vi "Doe_Julabo_Control.vi"(0 "Julabo CF41 VISA":refnum<visa-resource-name>="COM3", 1 "Data Cluster In":T1={"Current DoE"=[], "SSI 1 Flow Rate"=0.0, "SSI 2 Flow Rate"=0.0, "FLOM 1 Flow Rate"=0.0, "FLOM 2 Flow Rate"=0.0, "Pumps Running?"=FALSE, "Boolean 2"=FALSE, "Boolean 3"=FALSE, "Boolean 4"=FALSE, "At Equilibrium?"=FALSE, "Script Running?"=FALSE, "Current Script Iteration"=0.0, "Total Script Iterations"=0.0, "FLOM Pumps VISA"="COM2", "SSI 1 Pump VISA"="COM76", "SSI 2 Pump VISA"="COM74", "Huber Unistat VISA"="COM1", "SSI 3 Pump VISA"="COM76", "SSI 4 Pump VISA"="COM76", "SSI 4 Flow Rate"=0.0, "SSI 3 Flow Rate"=0.0, "Flow Meter 1 Rate "=0.0, "Flow Meter 2 Rate"=0.0, "Flow Meter 3 Rate"=0.0, "Flow Meter 4 Rate"=0.0, "SSI 1 Flow Setpoint"=0.0, "SSI 2 Flow Setpoint"=0.0, "SSI 3 Flow Setpoint"=0.0, "SSI 4 Flow Setpoint"=0.0, "Temperature Setpoint"=0.0, "Flow meter 3 COM"=17, "Flow meter 5 COM"=18, "Flow meter 4 COM"=19, "Flow meter 2 COM"=16, "Flow meter 1 COM"=15, "Unit"=enum."PSI", "Pressure COM"="COM6", "Julabo Setpoint"=0.0, "Julabo Control"=enum."Internal", "Overtemp"=50.0, "Subtemp"=-20.0, "HeatMax"=50, "CoolMax"=-100, "InternMax"=50.0, "InternMin"=0.0, "Upper Bandlimit"=100.0, "Lower Bandlimit"=0.0, "Julabo CF41 VISA"="COM3", "Xp (0.6K) Int"=0.6, "Tn (3s) Int"=3, "Tv (0s) Int"=0, "Dynamic (0: aperiodic) Int"=enum."aperiodic", "Xp (0.6K) Ext"=0.6, "Tn (3s) Ext"=3, "Tv (0s) Ext"=0, "XpU (0.6K) Ext"=0.6} {"XpU (0.6K) Ext" min=0.1 max=99.9; "Tv (0s) Ext" max=999; "Tn (3s) Ext" min=3 max=9999; "Xp (0.6K) Ext" min=0.1 max=99.9; "Tv (0s) Int" max=999; "Tn (3s) Int" min=3 max=9999; "Xp (0.6K) Int" min=0.1 max=99.9; "Lower Bandlimit" min=0.0 max=200.0; "Upper Bandlimit" min=0.0 max=200.0; "InternMin" format="%.2f"; "InternMax" format="%.2f"; "CoolMax" min=-100 max=0; "HeatMax" max=100; "Subtemp" format="%.2f"; "Overtemp" format="%.2f"; "Julabo Setpoint" format="%.2f"; "Current DoE" format="%0.3f"}, 5 "Serial Configuration":T4={"Baud Rate"=4800, "Parity"=2, "Data Bits"=7, "Stop Bits"=10, "Flow Control"=2} {"Flow Control" items=["None", "XON/XOFF", "RTS/CTS", "XON/XOFF & RTS/CTS", "DTR/DSR", "XON/XOFF & DTR/DSR"]; "Stop Bits" items=["1.0"=10, "1.5"=15, "2.0"=20]; "Data Bits" items=["7"=7, "8"=8]; "Parity" items=["None", "Odd", "Even", "Mark", "Space"]; "Baud Rate" items=["300"=300, "600"=600, "1200"=1200, "2400"=2400, "4800"=4800, "9600"=9600, "19200"=19200]}, 7 "RS485-Address (128: RS232)":u32=128, 9 "ID Query? (T: Yes)":bool=TRUE, 11 "ReadCycle":i32=1000) -> (4 "Data Cluster Out":T1={"Current DoE"=[], "SSI 1 Flow Rate"=0.0, "SSI 2 Flow Rate"=0.0, "FLOM 1 Flow Rate"=0.0, "FLOM 2 Flow Rate"=0.0, "Pumps Running?"=FALSE, "Boolean 2"=FALSE, "Boolean 3"=FALSE, "Boolean 4"=FALSE, "At Equilibrium?"=FALSE, "Script Running?"=FALSE, "Current Script Iteration"=0.0, "Total Script Iterations"=0.0, "FLOM Pumps VISA"="COM2", "SSI 1 Pump VISA"="COM76", "SSI 2 Pump VISA"="COM74", "Huber Unistat VISA"="COM1", "SSI 3 Pump VISA"="COM76", "SSI 4 Pump VISA"="COM76", "SSI 4 Flow Rate"=0.0, "SSI 3 Flow Rate"=0.0, "Flow Meter 1 Rate "=0.0, "Flow Meter 2 Rate"=0.0, "Flow Meter 3 Rate"=0.0, "Flow Meter 4 Rate"=0.0, "SSI 1 Flow Setpoint"=0.0, "SSI 2 Flow Setpoint"=0.0, "SSI 3 Flow Setpoint"=0.0, "SSI 4 Flow Setpoint"=0.0, "Temperature Setpoint"=0.0, "Flow meter 3 COM"=17, "Flow meter 5 COM"=18, "Flow meter 4 COM"=19, "Flow meter 2 COM"=16, "Flow meter 1 COM"=15, "Unit"=enum."PSI", "Pressure COM"="COM6", "Julabo Setpoint"=0.0, "Julabo Control"=enum."Internal", "Overtemp"=50.0, "Subtemp"=-20.0, "HeatMax"=50, "CoolMax"=-100, "InternMax"=50.0, "InternMin"=0.0, "Upper Bandlimit"=100.0, "Lower Bandlimit"=0.0, "Julabo CF41 VISA"="COM3", "Xp (0.6K) Int"=0.6, "Tn (3s) Int"=3, "Tv (0s) Int"=0, "Dynamic (0: aperiodic) Int"=enum."aperiodic", "Xp (0.6K) Ext"=0.6, "Tn (3s) Ext"=3, "Tv (0s) Ext"=0, "XpU (0.6K) Ext"=0.6} {"XpU (0.6K) Ext" min=0.1 max=99.9; "Tv (0s) Ext" max=999; "Tn (3s) Ext" min=3 max=9999; "Xp (0.6K) Ext" min=0.1 max=99.9; "Tv (0s) Int" max=999; "Tn (3s) Int" min=3 max=9999; "Xp (0.6K) Int" min=0.1 max=99.9; "Lower Bandlimit" min=0.0 max=200.0; "Upper Bandlimit" min=0.0 max=200.0; "InternMin" format="%.2f"; "InternMax" format="%.2f"; "CoolMax" min=-100 max=0; "HeatMax" max=100; "Subtemp" format="%.2f"; "Overtemp" format="%.2f"; "Julabo Setpoint" format="%.2f"; "Current DoE" format="%0.3f"}, 6 "Internal Temp":dbl format="%.2f", 8 "External Temp":dbl format="%.2f", 15 "device error out":errorcluster)   [LabVIEW 2015, in "JULABO DeviceDriver.lvlib"]
doc: "Advanced event triggered example"
uses:
  <instrlib>/JULABO DeviceDriver/JULABO DeviceDriver.lvlib
  <instrlib>/JULABO DeviceDriver/Examples/Julabo Serial Control.ctl
  --Controls and TypeDefs--/DoE_Control_Cluster.ctl
panel:
  out "error out 2":errorcluster caption="error out"
  out "error out":errorcluster
  in  "Registerkartenelement":T2(tab)
  out "Safety Temp":dbl
  out "Excess Temp Protection":dbl
  in  "Control":enum16{"Internal", "External"}(ring)
  in  "Setpoint":dbl format="%.2f"
  out "Power":i8(slide) scale=-100.0..100.0
  out "Diagram":T3(graph)
  in  "StartStop":bool
  in  "btnAdjustInternalTempLimits":bool
  in  "btnAdjustBandLimits":bool
  in  "btnAdjustCapacityLevels":bool
  in  "btnAdjustWarningLevels":bool
  in  "Upper Bandlimit":dbl=100.0 min=0.0 max=200.0
  in  "Lower Bandlimit":dbl min=0.0 max=200.0
  in  "InternMin":dbl format="%.2f"
  in  "InternMax":dbl=50.0 format="%.2f"
  in  "CoolMax":i8=-100 min=-100 max=0
  in  "HeatMax":u8=50 max=100
  in  "Subtemp":dbl=-20.0 format="%.2f"
  in  "Overtemp":dbl=50.0 format="%.2f"
  in  "Tv (0s) 2":u16 max=999
  in  "Tn (3s) 2":u16=3 min=3 max=9999
  in  "Xp (0.6K) 2":dbl=0.6 min=0.1 max=99.9
  in  "btnAdjustExternalControlParams":bool
  in  "XpU (0.6K)":dbl=0.6 min=0.1 max=99.9
  in  "Dynamic (0: aperiodic)":enum16{"aperiodic", "standard"}(ring)
  in  "btnAdjustInternalControlParams":bool
  in  "Tv (0s)":u16 max=999
  in  "Tn (3s)":u16=3 min=3 max=9999
  in  "Xp (0.6K)":dbl=0.6 min=0.1 max=99.9
  in  "Stopp":bool
  in  "Reset / Default (T: Both)":bool=TRUE
  # "1. Select the COM-Port and adjust the serial\nconfiguration for your instrument\n2. Adjust the Read cycle\n3. Start the VI by pressing the \"Start\" -Button\n( Arrow button on the top-left corner)\n4. To stop the execution press the \"Stop\" button"
  # "Julabo"
  # "Limits"
  # "PID Control Parameters"
  # "Julabo"
  # "Limits"
  # "PID Control Parameters"
  # "Internal parameters"
  # "External parameters"
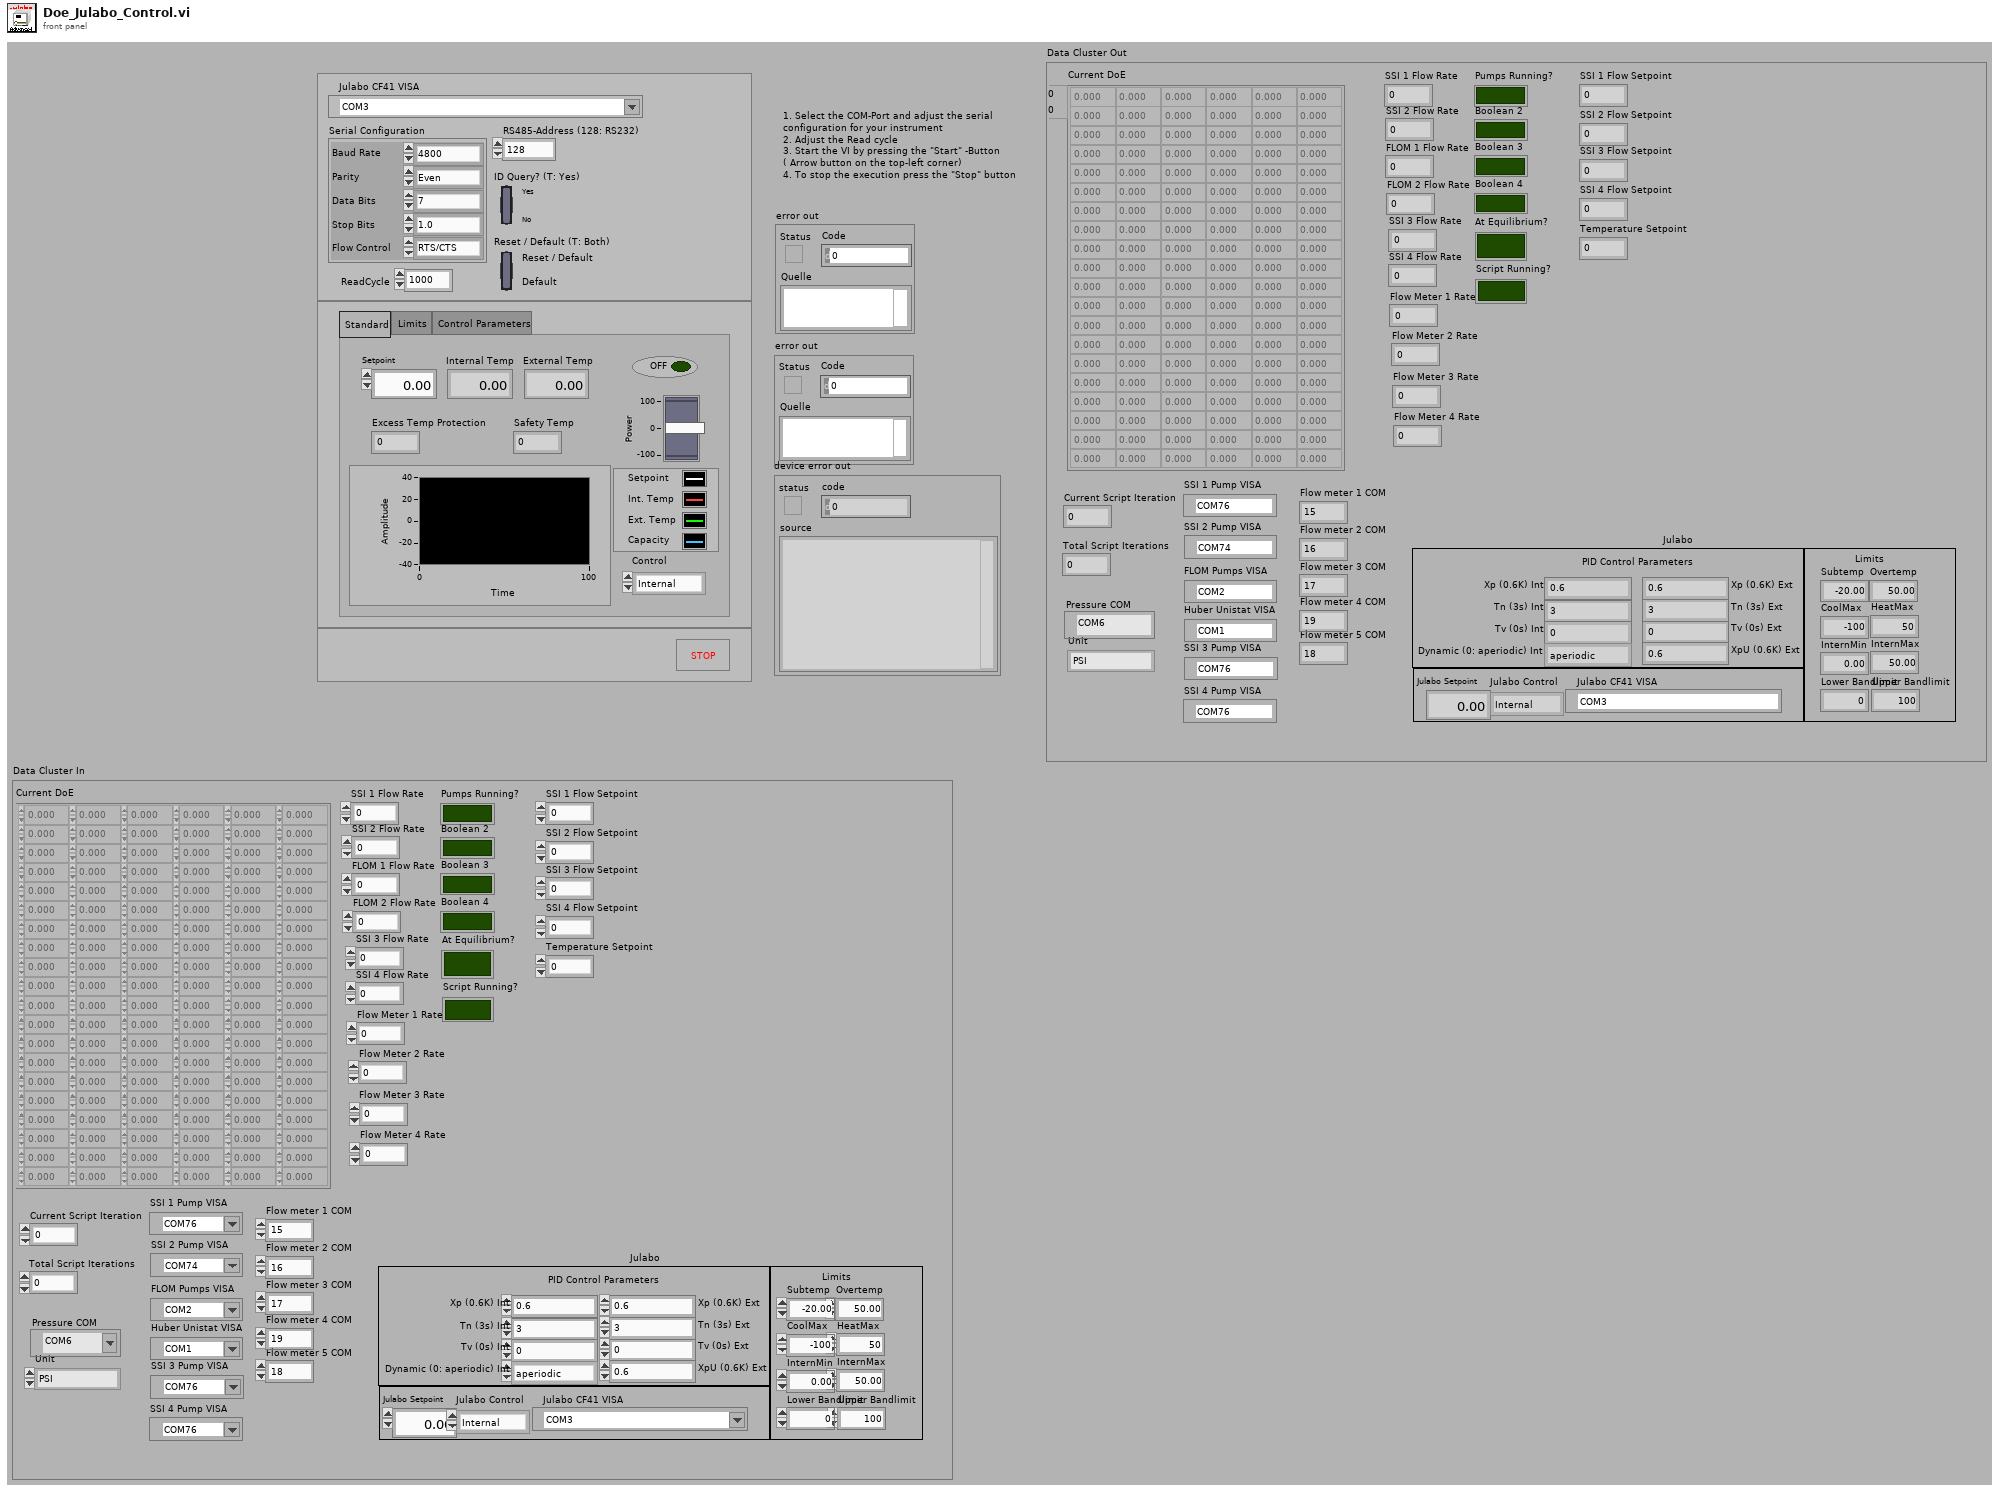
[diagram p1: front panel]
types:
  T1 = typedef "DoE_Control_Cluster.ctl" = cluster{"Current DoE":dbl[][], "SSI 1 Flow Rate":dbl, "SSI 2 Flow Rate":dbl, "FLOM 1 Flow Rate":dbl, "FLOM 2 Flow Rate":dbl, "Pumps Running?":bool, "Boolean 2":bool, "Boolean 3":bool, "Boolean 4":bool, "At Equilibrium?":bool, "Script Running?":bool, "Current Script Iteration":dbl, "Total Script Iterations":dbl, "FLOM Pumps VISA":refnum<visa-resource-name>, "SSI 1 Pump VISA":refnum<visa-resource-name>, "SSI 2 Pump VISA":refnum<visa-resource-name>, "Huber Unistat VISA":refnum<visa-resource-name>, "SSI 3 Pump VISA":refnum<visa-resource-name>, "SSI 4 Pump VISA":refnum<visa-resource-name>, "SSI 4 Flow Rate":dbl, "SSI 3 Flow Rate":dbl, "Flow Meter 1 Rate ":dbl, "Flow Meter 2 Rate":dbl, "Flow Meter 3 Rate":dbl, "Flow Meter 4 Rate":dbl, "SSI 1 Flow Setpoint":dbl, "SSI 2 Flow Setpoint":dbl, "SSI 3 Flow Setpoint":dbl, "SSI 4 Flow Setpoint":dbl, "Temperature Setpoint":dbl, "Flow meter 3 COM":u16, "Flow meter 5 COM":u16, "Flow meter 4 COM":u16, "Flow meter 2 COM":u16, "Flow meter 1 COM":u16, "Unit":enum16{"PSI", "Bar", "cm H2O", "ft H2O", "hectoPascal", "in Hg", "in H2O", "kiloPascal", "milliBar", "mmHg", "MegaPascal", "Numeric Pressure"}, "Pressure COM":refnum<visa-resource-name>, "Julabo Setpoint":dbl, "Julabo Control":enum16{"Internal", "External"}, "Overtemp":dbl, "Subtemp":dbl, "HeatMax":u8, "CoolMax":i8, "InternMax":dbl, "InternMin":dbl, "Upper Bandlimit":dbl, "Lower Bandlimit":dbl, "Julabo CF41 VISA":refnum<visa-resource-name>, "Xp (0.6K) Int":dbl, "Tn (3s) Int":u16, "Tv (0s) Int":u16, "Dynamic (0: aperiodic) Int":enum16{"aperiodic", "standard"}, "Xp (0.6K) Ext":dbl, "Tn (3s) Ext":u16, "Tv (0s) Ext":u16, "XpU (0.6K) Ext":dbl}
  T2 = enum32{"Standard", "Limits", "Control Parameters"}
  T3 = cluster{"Setpoint (out)":dbl, "InternalTemp (out)":dbl, "ExternalTemp (out)":dbl, "Capacity (out)":i8}
  T4 = typedef "Julabo Serial Control.ctl" = cluster{"Baud Rate":u32, "Parity":u16, "Data Bits":u16, "Stop Bits":u16, "Flow Control":u16}
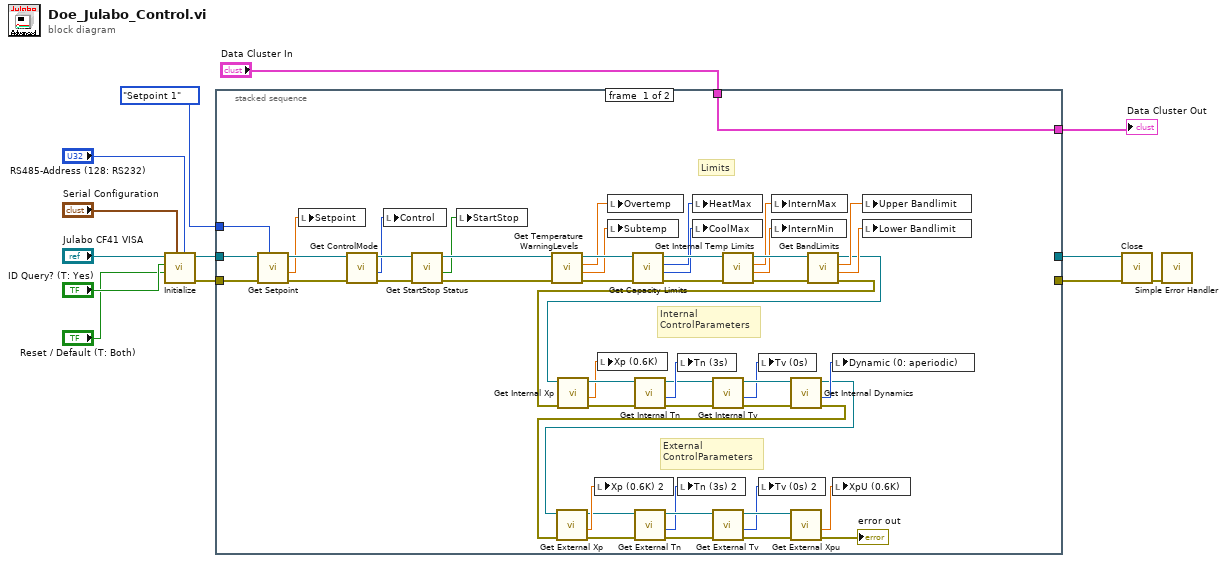
[diagram p0: block diagram]
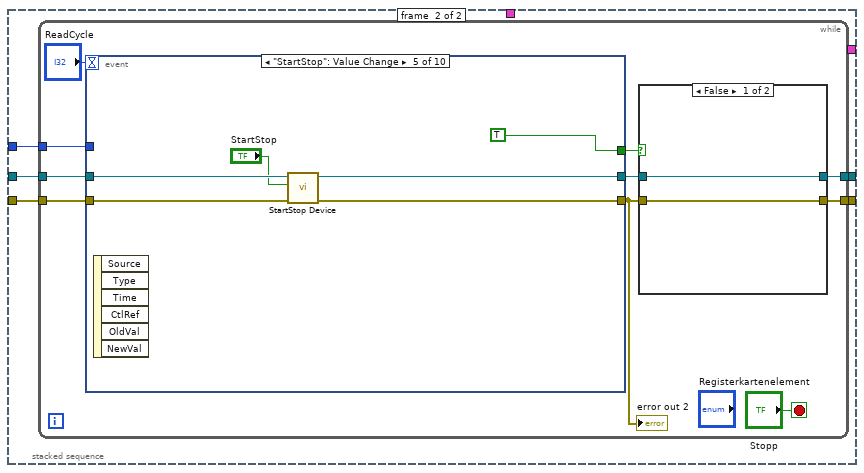
[diagram p2: hidden frame]
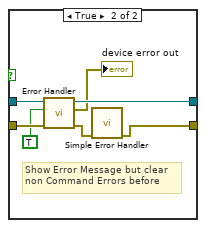
[diagram p3: hidden frame]
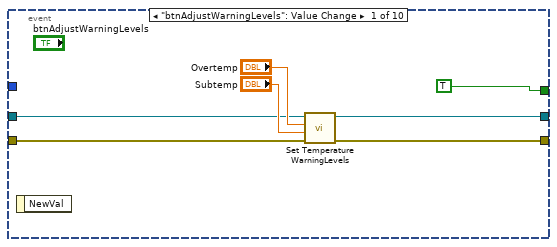
[diagram p4: hidden frame]
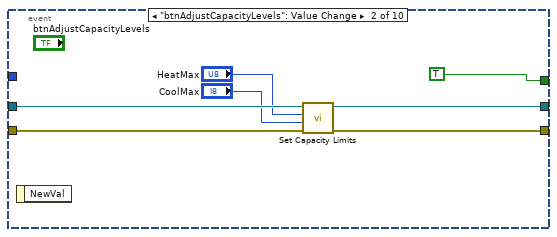
[diagram p5: hidden frame]
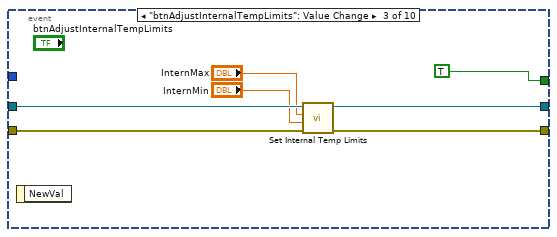
[diagram p6: hidden frame]
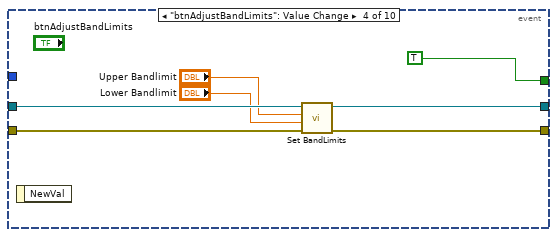
[diagram p7: hidden frame]
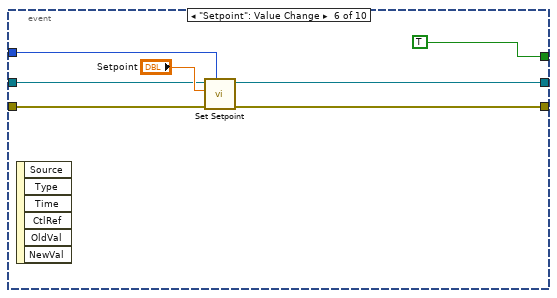
[diagram p8: hidden frame]
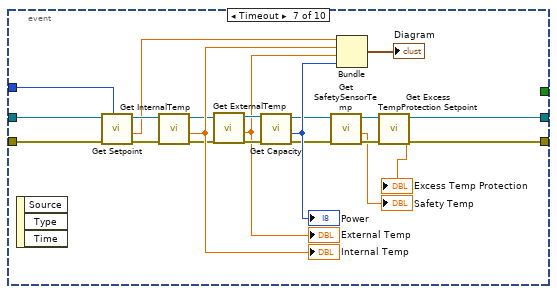
[diagram p9: hidden frame]
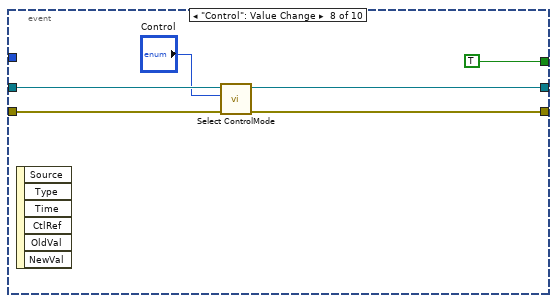
[diagram p10: hidden frame]
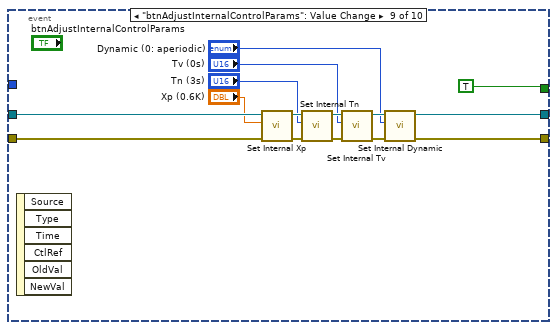
[diagram p11: hidden frame]
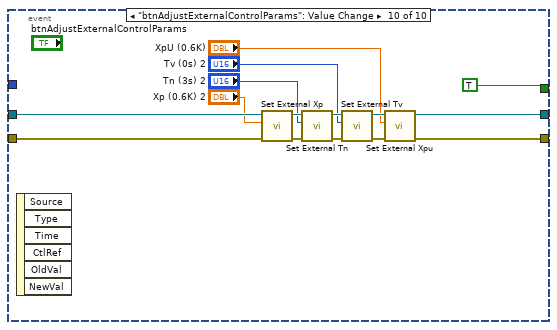
[diagram p12: hidden frame]
diagram:
  n1 = call <instrlib>:"Initialize.vi"("RS485-Address (128: RS232)"="RS485-Address (128: RS232)", "Serial Configuration"="Serial Configuration", "Reset / Default (T: Both)"="Reset / Default (T: Both)", "ID Query? (T: Yes)"="ID Query? (T: Yes)", "VISA resource name"="Julabo CF41 VISA") -> ("error out"=w6:errorcluster, "VISA resource name out"=w7:refnum<visa-resource-name>)  [unwired: 5 in]
  n2 = stacked-sequence {
    tunnel: w7 -> [w20 w70]
    tunnel: w6 -> [w19 w69]
    tunnel: [_ w68] -> w5
    tunnel: [_ w67] -> w4
    tunnel: enum16{"Setpoint 1", "Setpoint 2", "Setpoint 3"}."Setpoint 1" ("Setpointindex") -> [w16 w66]
    tunnel: "Data Cluster In" -> [w14 _]
    tunnel: [w14 _] -> w1
    frame #0 {
      # "External\nControlParameters"
      # "Internal\nControlParameters"
      # "Limits"
      n3 = call <instrlib>:"Get Setpoint.vi"("Setpointindex"=w16, "error in (no error)"=w19, "VISA resource name"=w20) -> ("error out"=w17:errorcluster, "Setpoint (out)"=w15:dbl, "VISA resource name out"=w18:refnum<visa-resource-name>)  [unwired: 6 in]
      n4 = local write "Setpoint"(w15) -> ()
      n5 = call <instrlib>:"Get ControlMode.vi"("error in"=w17, "VISA resource name in"=w18) -> ("error out"=w22:errorcluster, "Control (out)"=w26:enum16{"Internal", "External"}, "VISA resource name out"=w27:refnum<visa-resource-name>)  [unwired: 7 in]
      n6 = local write "Control"(w26) -> ()
      n7 = call <instrlib>:"Get StartStop Status.vi"("error in"=w22, "VISA resource name in"=w27) -> ("error out"=w21:errorcluster, "Status"=w23:bool, "VISA resource name out"=w24:refnum<visa-resource-name>)  [unwired: 7 in]
      n8 = local write "StartStop"(w23) -> ()
      n9 = call <instrlib>:"Get Temperature WarningLevels.vi"("error in (no error)"=w21, "VISA resource name"=w24) -> ("error out"=w62:errorcluster, "Subtemp (out)"=w53:dbl, "Overtemp (out)"=w52:dbl, "VISA resource name out"=w65:refnum<visa-resource-name>)  [unwired: 2 in]
      n10 = local write "Overtemp"(w52) -> ()
      n11 = local write "Subtemp"(w53) -> ()
      n12 = call <instrlib>:"Get Capacity Limits.vi"("error in (no error)"=w62, "VISA resource name"=w65) -> ("error out"=w61:errorcluster, "Maximum cooling capacity(out)"=w55:i8, "Maximum heating capacity(out)"=w54:u8, "VISA resource name out"=w64:refnum<visa-resource-name>)  [unwired: 2 in]
      n13 = local write "HeatMax"(w54) -> ()
      n14 = local write "CoolMax"(w55) -> ()
      n15 = call <instrlib>:"Get Internal Temp Limits.vi"("error in (no error)"=w61, "VISA resource name"=w64) -> ("error out"=w60:errorcluster, "IntMin (out)"=w57:dbl, "IntMax (out)"=w56:dbl, "VISA resource name out"=w63:refnum<visa-resource-name>)  [unwired: 2 in]
      n16 = local write "InternMax"(w56) -> ()
      n17 = local write "InternMin"(w57) -> ()
      n18 = call <instrlib>:"Get BandLimits.vi"("error in (no error)"=w60, "VISA resource name"=w63) -> ("error out"=w40:errorcluster, "LowerBand (out)"=w59:dbl, "UpperBand (out)"=w58:dbl, "VISA resource name out"=w41:refnum<visa-resource-name>)  [unwired: 2 in]
      n19 = call <instrlib>:"Get Internal Xp.vi"("error in"=w40, "VISA resource name in"=w41) -> ("error out"=w43:errorcluster, "InternalXp (out)"=w42:dbl, "VISA resource name out"=w44:refnum<visa-resource-name>)  [unwired: 7 in]
      n20 = local write "Xp (0.6K)"(w42) -> ()
      n21 = call <instrlib>:"Get Internal Tn.vi"("error in"=w43, "VISA resource name in"=w44) -> ("error out"=w45:errorcluster, "InternalTn (out)"=w51:u16, "VISA resource name out"=w46:refnum<visa-resource-name>)  [unwired: 7 in]
      n22 = local write "Tn (3s)"(w51) -> ()
      n23 = call <instrlib>:"Get Internal Tv.vi"("error in"=w45, "VISA resource name in"=w46) -> ("error out"=w48:errorcluster, "InternalTv (out)"=w47:u16, "VISA resource name out"=w49:refnum<visa-resource-name>)  [unwired: 7 in]
      n24 = local write "Tv (0s)"(w47) -> ()
      n25 = call <instrlib>:"Get Internal Dynamics.vi"("error in"=w48, "VISA resource name in"=w49) -> ("error out"=w32:errorcluster, "Dynamic (out)"=w50:enum16{"aperiodic", "standard"}, "VISA resource name out"=w31:refnum<visa-resource-name>)  [unwired: 7 in]
      n26 = call <instrlib>:"Get External Xp.vi"("error in"=w32, "VISA resource name in"=w31) -> ("error out"=w35:errorcluster, "ExternalXp (out)"=w34:dbl, "VISA resource name out"=w30:refnum<visa-resource-name>)  [unwired: 7 in]
      n27 = local write "Xp (0.6K) 2"(w34) -> ()
      n28 = call <instrlib>:"Get External Tn.vi"("error in"=w35, "VISA resource name in"=w30) -> ("error out"=w39:errorcluster, "ExternalTn (out)"=w29:u16, "VISA resource name out"=w38:refnum<visa-resource-name>)  [unwired: 7 in]
      n29 = local write "Tn (3s) 2"(w29) -> ()
      n30 = call <instrlib>:"Get External Tv.vi"("error in"=w39, "VISA resource name in"=w38) -> ("error out"=w37:errorcluster, "ExternalTv (out)"=w28:u16, "VISA resource name out"=w36:refnum<visa-resource-name>)  [unwired: 7 in]
      n31 = local write "Tv (0s) 2"(w28) -> ()
      n32 = call <instrlib>:"Get External Xpu.vi"("error in"=w37, "VISA resource name in"=w36) -> ("error out"=→"error out":errorcluster, "ExternalXpu (out)"=w33:dbl)  [unwired: 7 in, 1 out]
      n33 = local write "Dynamic (0: aperiodic)"(w50) -> ()
      n34 = local write "XpU (0.6K)"(w33) -> ()
      n35 = local write "Upper Bandlimit"(w58) -> ()
      n36 = local write "Lower Bandlimit"(w59) -> ()
    }
    frame #1 {
      n37 = while {
        tunnel: w70 -> [w80]
        tunnel: w69 -> [w79]
        tunnel: [w77] -> w67
        tunnel: [w76] -> w68
        tunnel: w66 -> [w72]
        stop <- "Stopp" stop-if-true
        n38 = event shown="[4] \"StartStop\": Value Change" {
          selector: _ -> [_ _ _ _ _ _ _ _ _ _]
          dyn-events: _ -> [_ _ _ _ _ _ _ _ _ _]
          timeout: "ReadCycle" -> [_ _ _ _ _ _ _ _ _ _]
          tunnel: [w91 w99 w109 w116 w120 w127 w137 w156 w162 w177] -> w78
          tunnel: [w90 w98 w108 w115 w121 w126 w136 w155 w160 w175] -> w71
          tunnel: w80 -> [w94 w103 w107 w113 w119 w129 w148 w158 w173 w188]
          tunnel: w79 -> [w93 w102 w106 w114 w122 w128 w147 w157 w172 w187]
          tunnel: [TRUE TRUE TRUE TRUE TRUE TRUE _ TRUE TRUE TRUE] -> w75
          tunnel: w72 -> [_ _ _ _ _ w124 w131 _ _ _]
          event "btnAdjustWarningLevels": Value Change {
            n39 = event-data() -> ()  [unwired: 1 in, 1 out]
            n40 = call <instrlib>:"Set Temperature WarningLevels.vi"("error in (no error)"=w93, "Subtemp (-20.00°C)"="Subtemp", "Overtemp (50.00°C)"="Overtemp", "VISA resource name"=w94) -> ("error out"=w90:errorcluster, "VISA resource name out"=w91:refnum<visa-resource-name>)  [unwired: 6 in]
          }
          event "btnAdjustCapacityLevels": Value Change {
            n41 = event-data() -> ()  [unwired: 1 in, 1 out]
            n42 = call <instrlib>:"Set Capacity Limits.vi"("error in (no error)"=w102, "Maximum cooling capacity(-100%)"="CoolMax", "Maximum heating capacity(100%)"="HeatMax", "VISA resource name"=w103) -> ("error out"=w98:errorcluster, "VISA resource name out"=w99:refnum<visa-resource-name>)  [unwired: 6 in]
          }
          event "btnAdjustInternalTempLimits": Value Change {
            n43 = event-data() -> ()  [unwired: 1 in, 1 out]
            n44 = call <instrlib>:"Set Internal Temp Limits.vi"("error in (no error)"=w106, "InternMin (-20.00 °C)"="InternMin", "InternMax (50.00 °C)"="InternMax", "VISA resource name"=w107) -> ("error out"=w108:errorcluster, "VISA resource name out"=w109:refnum<visa-resource-name>)  [unwired: 6 in]
          }
          event "btnAdjustBandLimits": Value Change {
            n45 = event-data() -> ()  [unwired: 1 in, 1 out]
            n46 = call <instrlib>:"Set BandLimits.vi"("error in (no error)"=w114, "Lower Bandlimit (200K)"="Lower Bandlimit", "Upper Bandlimit (200K)"="Upper Bandlimit", "VISA resource name"=w113) -> ("error out"=w115:errorcluster, "VISA resource name out"=w116:refnum<visa-resource-name>)  [unwired: 6 in]
          }
          event "StartStop": Value Change {
            n47 = event-data() -> ()  [unwired: 1 in, 6 out]
            n48 = call <instrlib>:"StartStop Device.vi"("error in (no error)"=w122, "Start/Stop (f:Stop)"="StartStop", "VISA resource name"=w119) -> ("error out"=w121:errorcluster, "VISA resource name out"=w120:refnum<visa-resource-name>)  [unwired: 7 in]
          }
          event "Setpoint": Value Change {
            n49 = event-data() -> ()  [unwired: 1 in, 6 out]
            n50 = call <instrlib>:"Set Setpoint.vi"("Setpointindex (Setpoint1: Default)"=w124, "error in (no error)"=w128, "newSetpoint (20.00°C)"="Setpoint", "VISA resource name"=w129) -> ("error out"=w126:errorcluster, "VISA resource name out"=w127:refnum<visa-resource-name>)  [unwired: 6 in]
          }
          event Timeout {
            n51 = event-data() -> ()  [unwired: 1 in, 3 out]
            n52 = call <instrlib>:"Get Setpoint.vi"("Setpointindex"=w131, "error in (no error)"=w147, "VISA resource name"=w148) -> ("error out"=w152:errorcluster, "Setpoint (out)"=w146:dbl, "VISA resource name out"=w151:refnum<visa-resource-name>)  [unwired: 6 in]
            n53 = call <instrlib>:"Get InternalTemp.vi"("error in (no error)"=w152, "VISA resource name"=w151) -> ("error out"=w144:errorcluster, "InternalTemp (out)"=w149:dbl, "VISA resource name out"=w145:refnum<visa-resource-name>)  [unwired: 7 in]
            "Internal Temp" <- w149
            n54 = call <instrlib>:"Get ExternalTemp.vi"("error in (no error)"=w144, "VISA resource name"=w145) -> ("error out"=w142:errorcluster, "ExternalTemp (out)"=w140:dbl, "VISA resource name out"=w143:refnum<visa-resource-name>)  [unwired: 6 in, 1 out]
            "External Temp" <- w140
            n55 = call <instrlib>:"Get Capacity.vi"("error in (no error)"=w142, "VISA resource name"=w143) -> ("error out"=w134:errorcluster, "Capacity (out)"=w141:i8, "VISA resource name out"=w139:refnum<visa-resource-name>)  [unwired: 7 in]
            "Power" <- w141
            n56 = call <instrlib>:"Get SafetySensorTemp.vi"("error in (no error)"=w134, "VISA resource name"=w139) -> ("error out"=w135:errorcluster, "Safetytemp (out)"=→"Safety Temp":dbl, "VISA resource name out"=w138:refnum<visa-resource-name>)  [unwired: 7 in]
            n57 = Bundle("Setpoint (out)"=w146, "InternalTemp (out)"=w149, "ExternalTemp (out)"=w140, "Capacity (out)"=w141) -> (→"Diagram":T3)  [unwired: 1 in]
            n58 = call <instrlib>:"Get Excess TempProtection Setpoint.vi"("error in (no error)"=w135, "VISA resource name"=w138) -> ("error out"=w136:errorcluster, "ExcessTempProtection(out)"=→"Excess Temp Protection":dbl, "VISA resource name out"=w137:refnum<visa-resource-name>)  [unwired: 7 in]
          }
          event "Control": Value Change {
            n59 = event-data() -> ()  [unwired: 1 in, 6 out]
            n60 = call <instrlib>:"Select ControlMode.vi"("error in (no error)"=w157, "Control (0: Internal)"="Control", "VISA resource name"=w158) -> ("error out"=w155:errorcluster, "VISA resource name out"=w156:refnum<visa-resource-name>)  [unwired: 7 in]
          }
          event "btnAdjustInternalControlParams": Value Change {
            n61 = event-data() -> ()  [unwired: 1 in, 6 out]
            n62 = call <instrlib>:"Set Internal Xp.vi"("error in (no error)"=w172, "Xp (0.6K)"="Xp (0.6K)", "VISA resource name"=w173) -> ("error out"=w169:errorcluster, "VISA resource name out"=w168:refnum<visa-resource-name>)  [unwired: 7 in]
            n63 = call <instrlib>:"Set Internal Tn.vi"("error in (no error)"=w169, "Tn (3s)"="Tn (3s)", "VISA resource name"=w168) -> ("error out"=w171:errorcluster, "VISA resource name out"=w170:refnum<visa-resource-name>)  [unwired: 7 in]
            n64 = call <instrlib>:"Set Internal Tv.vi"("error in (no error)"=w171, "Tv (0s)"="Tv (0s)", "VISA resource name"=w170) -> ("error out"=w161:errorcluster, "VISA resource name out"=w164:refnum<visa-resource-name>)  [unwired: 7 in]
            n65 = call <instrlib>:"Set Internal Dynamic.vi"("error in (no error)"=w161, "Dynamic (0: aperiodic)"="Dynamic (0: aperiodic)", "VISA resource name"=w164) -> ("error out"=w160:errorcluster, "VISA resource name out"=w162:refnum<visa-resource-name>)  [unwired: 7 in]
          }
          event "btnAdjustExternalControlParams": Value Change {
            n66 = event-data() -> ()  [unwired: 1 in, 6 out]
            n67 = call <instrlib>:"Set External Xp.vi"("error in (no error)"=w187, "Xp (0.6K)"="Xp (0.6K) 2", "VISA resource name"=w188) -> ("error out"=w184:errorcluster, "VISA resource name out"=w183:refnum<visa-resource-name>)  [unwired: 7 in]
            n68 = call <instrlib>:"Set External Tn.vi"("error in (no error)"=w184, "Tn (3s)"="Tn (3s) 2", "VISA resource name"=w183) -> ("error out"=w186:errorcluster, "VISA resource name out"=w185:refnum<visa-resource-name>)  [unwired: 7 in]
            n69 = call <instrlib>:"Set External Tv.vi"("error in (no error)"=w186, "Tv (0s)"="Tv (0s) 2", "VISA resource name"=w185) -> ("error out"=w176:errorcluster, "VISA resource name out"=w179:refnum<visa-resource-name>)  [unwired: 7 in]
            n70 = call <instrlib>:"Set External Xpu.vi"("error in (no error)"=w176, "XpU (0.6K)"="XpU (0.6K)", "VISA resource name"=w179) -> ("error out"=w175:errorcluster, "VISA resource name out"=w177:refnum<visa-resource-name>)  [unwired: 7 in]
          }
        }
        "error out 2" <- w71
        n71 = case shown="False" w75 {
          tunnel: w78 -> [w82 w87]
          tunnel: [w82 w85] -> w77
          tunnel: w71 -> [w81 w88]
          tunnel: [w81 w89] -> w76
          frame False {
          }
          frame True {
            # "Show Error Message but clear\nnon Command Errors before"
            n72 = call <instrlib>:"Error Handler.vi"("error in (no error)"=w88, "ClearDeviceError (false)"=TRUE, "VISA resource name"=w87) -> ("error out"=w86:errorcluster, "device error out"=→"device error out":errorcluster, "VISA resource name out"=w85:refnum<visa-resource-name>)  [unwired: 5 in, 1 out]
            n73 = call <vilib>:"Simple Error Handler.vi"("error in (no error)"=w86) -> ("error out"=w89:errorcluster)  [unwired: 4 in, 4 out]
          }
        }
      }
    }
  }
  "Data Cluster Out" <- w1
  n74 = call <instrlib>:"Close.vi"("error in (no error)"=w5, "VISA resource name"=w4) -> ("error out"=w11:errorcluster)  [unwired: 9 in]
  n75 = call <vilib>:"Simple Error Handler.vi"("error in (no error)"=w11) -> ()  [unwired: 4 in, 5 out]
